vi "SubVI_timeconstant_lowpass_filter.vi"(1 "Init/reset":bool, 2 "Ts [s]":dbl=0.1 caption="Time-step, Ts [s]" min=0.0, 3 "Tf [s]":dbl=5.0 caption="Filter time-constant, Tf [s]" min=0.0, 4 "Filter_input":dbl=20.0) -> (0 "Filter_output":dbl=20.0)   [LabVIEW 2022 SP3]
panel:
  # "Finn Haugen (finn.haugen@hit.no)"
  # "20. October 2008"
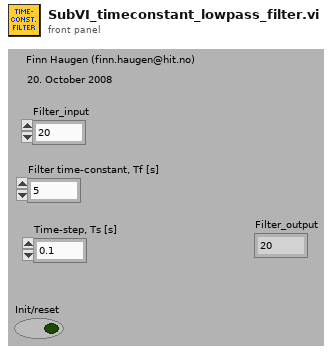
[diagram p1: front panel]
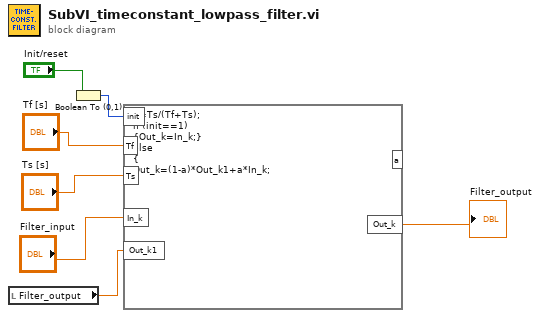
[diagram p0: block diagram]
diagram:
  n1 = local read "Filter_output"() -> (w3:dbl)
  n2 = Boolean To (0,1)(Boolean="Init/reset") -> (0, 1=w2:i16)
  n3 = formula code="a=Ts/(Tf+Ts);\nif (init==1)\n{Out_k=In_k;}\nelse\n{\nOut_k=(1-a)*Out_k1+a*In_k;\n}"("Tf"="Tf [s]", "Ts"="Ts [s]", "Out_k1"=w3, "In_k"="Filter_input", "init"=w2) -> ("Out_k"=→"Filter_output":dbl)  [unwired: 1 out]
